vi "Write Enum.vi"(8 "error in (no error)":errorcluster, 10 "Enum":bool, 11 "baseClass in":refnum<class "baseClass.lvclass">) -> (0 "error out":errorcluster, 3 "baseClass out":refnum<class "baseClass.lvclass">)   [LabVIEW 2013, in "baseClass.lvclass"]
uses:
  baseClass.lvclass
  baseClass.lvclass/baseClass.ctl
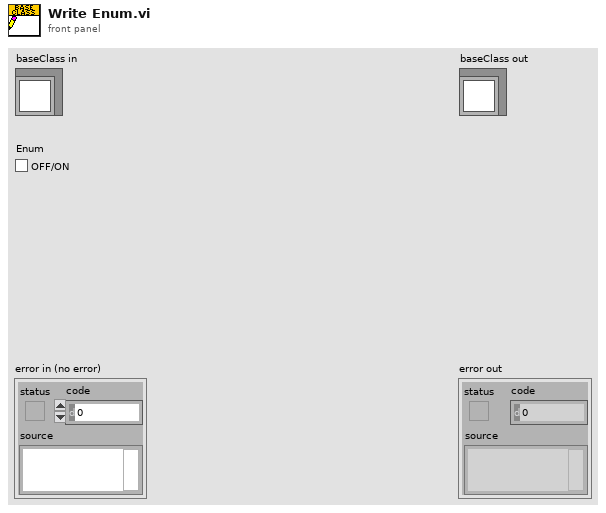
[diagram p1: front panel]
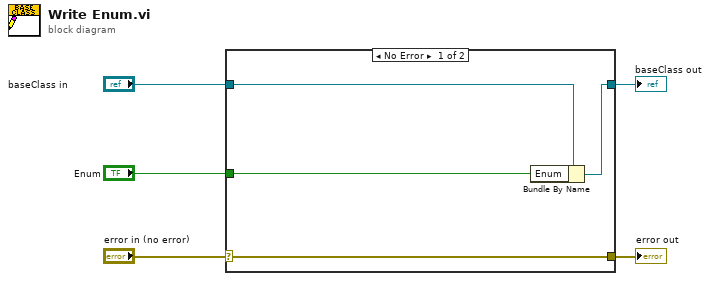
[diagram p0: block diagram]
diagram:
  n1 = case shown="No Error" "error in (no error)" {
    selector: "error in (no error)" -> [w9 w10]
    tunnel: [w9 w10] -> w4
    tunnel: [w7 w11] -> w2
    tunnel: "baseClass in" -> [w8 w11]
    tunnel: "Enum" -> [w6 _]
    frame No Error {
      n2 = Bundle By Name(cluster=w8, "Enum"=w6) -> (w7:refnum<class "baseClass.lvclass">)
    }
    frame Error {
    }
  }
  "error out" <- w4
  "baseClass out" <- w2
